vi "setUpdateOnline.vi"(8 "error in (no error)":errorcluster, 10 "onlineUpdate":timestamp, 11 "reference in":refnum<class "Notification Controller.lvclass">) -> (0 "error out":errorcluster, 3 "reference out":refnum<class "Notification Controller.lvclass">)   [LabVIEW 2014, in "Notification Controller.lvclass"]
uses:
  Notification Controller.lvclass
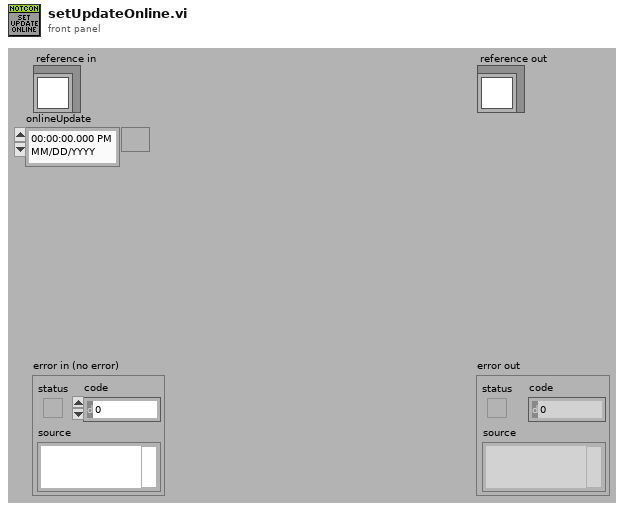
[diagram p1: front panel]
types:
  T1 = typedef "Notification Controller.lvclass/ObjectAttributesRef.ctl" = refnum<data-value>
  T2 = typedef "Notification Controller.lvclass/ObjectAttributes.ctl" = cluster{"MyAttribute":dbl, "items_data":string[][][], "items_notification_refs":refnum<class "itemsNotification.lvclass">[], "notifications_data_items":string[][], "items_nots?":bool, "devices_controller_ref":refnum<class "Devices Controller.lvclass">, "onlineUpdate":timestamp, "notController?":bool, "tracking_notification_ref":refnum<class "trackingNotification.lvclass">, "notifications_data_tracking":string[][], "tracking_parts_data":string[][], "tracking_nots?":bool, "index_tracking_not":i32[], "file_controller_ref":refnum<class "File Controller.lvclass">}
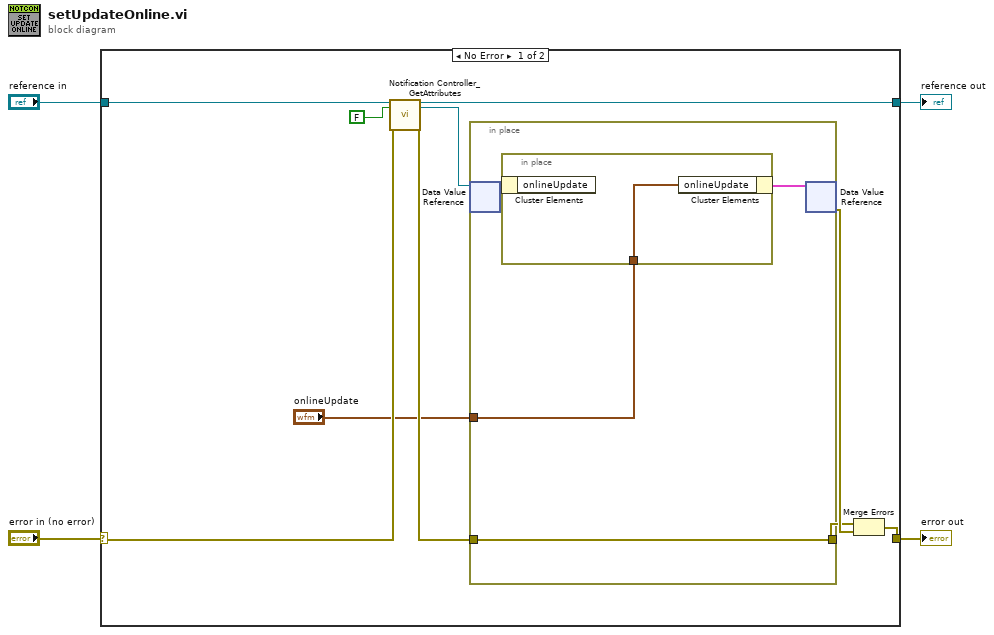
[diagram p0: block diagram]
diagram:
  n1 = case shown="No Error" "error in (no error)" {
    selector: "error in (no error)" -> [w9 w21]
    tunnel: [w14 w21] -> w3
    tunnel: [w7 w20] -> w1
    tunnel: "reference in" -> [w11 w20]
    frame No Error {
      n2 = call "Notification Controller_GetAttributes.vi"("reference in"=w11, "return data? (T)"=FALSE, "error in (no error)"=w9) -> ("reference out"=w7:refnum<class "Notification Controller.lvclass">, "attributes ref"=w6:T1, "error out"=w8:errorcluster)  [unwired: 13 in, 1 out]
      n3 = in-place {
        in-place-border: w8 -> [w16]
        in-place-border: [w16] -> w12
        in-place-border: "onlineUpdate" -> [w15]
        n4 = in-place-dvr #1(w6) -> (w17:T2)  [unwired: 1 out]
        n5 = in-place {
          in-place-border: w15 -> [w19]
          n6 = in-place-cluster #2(w17) -> ()  [unwired: 1 out]
          n7 = in-place-cluster #2("onlineUpdate"=w19) -> (w18:T2)
        }
        n8 = in-place-dvr #1(w18) -> (w13:errorcluster)  [unwired: 1 out]
      }
      n9 = Merge Errors(w12, w13) -> (w14:errorcluster)
    }
    frame Error {
    }
  }
  "error out" <- w3
  "reference out" <- w1
